vi "Configure.vi"(8 "error in (no error)":errorcluster, 9 "Eye Params":dbl[](array[numeric]), 11 "TrialBasedExperiment in":refnum<class "TrialBasedExperiment.lvclass">) -> (0 "error out":errorcluster, 3 "TrialBasedExperiment out":refnum<class "TrialBasedExperiment.lvclass">)   [LabVIEW 2011, in "TrialBasedExperiment.lvclass"]
uses:
  TrialBasedExperiment.lvclass
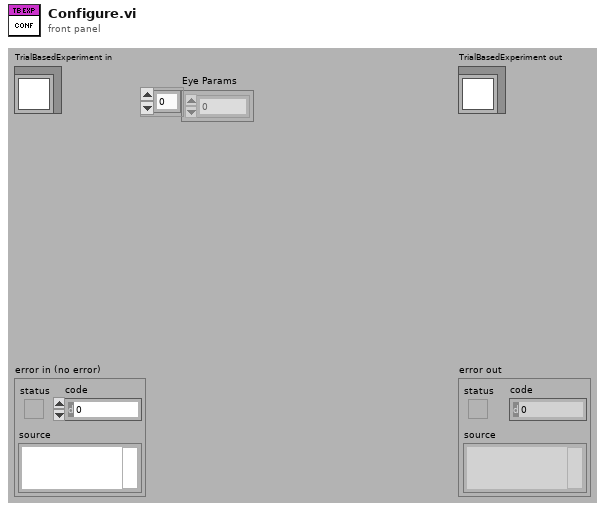
[diagram p1: front panel]
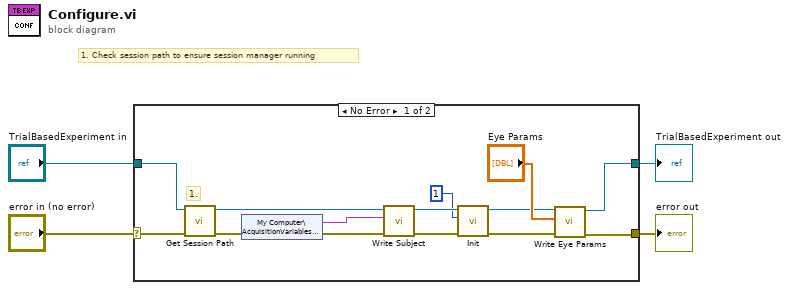
[diagram p0: block diagram]
diagram:
  # "1. Check session path to ensure session manager running"
  n1 = case shown="No Error" "error in (no error)" {
    selector: "error in (no error)" -> [w13 w20]
    tunnel: [w8 w20] -> w3
    tunnel: [w7 w19] -> w1
    tunnel: "TrialBasedExperiment in" -> [w15 w19]
    frame No Error {
      # "1."
      n2 = call-dynamic "Get Session Path.vi"("error in (no error)"=w13, "AcquistionObject in"=w15) -> ("error out"=w16:errorcluster, "AcquistionObject out"=w14:refnum<class "TrialBasedExperiment.lvclass">)  [unwired: 7 in, 1 out]
      n3 = shared-variable "My Computer\\AcquisitionVariables.lvlib\\Subject"(error in=w16) -> (w18:string, error out=w17:errorcluster)
      n4 = call-dynamic "Write Subject.vi"("error in (no error)"=w17, "Subject"=w18, "TrialBasedExperiment in"=w14) -> ("error out"=w12:errorcluster, "TrialBasedExperiment out"=w11:refnum<class "TrialBasedExperiment.lvclass">)  [unwired: 7 in]
      n5 = call-dynamic "Init.vi"("error in (no error)"=w12, "Channel"=i16 1, "TrialBasedExperiment in"=w11) -> ("error out"=w5:errorcluster, "TrialBasedExperiment out"=w6:refnum<class "TrialBasedExperiment.lvclass">)  [unwired: 7 in]
      n6 = call-dynamic "Write Eye Params.vi"("error in (no error)"=w5, "Eye Params"="Eye Params", "TrialBasedExperiment in"=w6) -> ("error out"=w8:errorcluster, "TrialBasedExperiment out"=w7:refnum<class "TrialBasedExperiment.lvclass">)  [unwired: 7 in]
    }
    frame Error {
    }
  }
  "error out" <- w3
  "TrialBasedExperiment out" <- w1
